vi "ALTS-2015 Scanner Driverv2.vi"(7 "Operation":T1, 8 "error in (no error)":errorcluster, 11 "Scanner 2?  (Scanner1)":bool) -> (0 "error out":errorcluster, 3 "Serial No":string)   [LabVIEW 2013]
doc: "Copyright © 2005, Soliton Technologies.\nAll rights reserved."
uses:
  <vilib>/Utility/file.llb/Read From Spreadsheet File (string).vi
  Controls/ALTS-2015 LV2GBL Options.ctl
  Controls/ALTS-2015 Scanner Driver Options.ctl
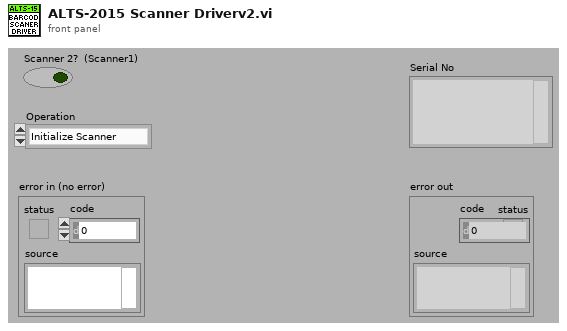
[diagram p1: front panel]
types:
  T1 = typedef "ALTS-2015 Scanner Driver Options.ctl" = enum16{"Initialize Scanner", "Read Scanner", "Close Scanner"}
  T2 = typedef "ALTS-2015 LV2GBL Options.ctl" = enum16{"Read all", "Write all"}
  T3 = typedef "ALTS-2015 INI Configuration Cluster.ctl" = cluster{"Application":cluster{"Rerun Count":i32, "Workorder No":string, "PLC Scanner":bool}, "Station Details":cluster{"Sensor Name 1":string, "Sensor Name 2":string, "Sensor Name 3":string, "Sensor Name 4":string, "Station1 Enable":bool, "Station2 Enable":bool, "Station3 Enable":bool, "Station4 Enable":bool}, "Database":cluster{"Database Connection Link":path, "Result Procedure":string, "User":string, "Password":string, "Prompt":bool, "Station 1 LT Result DB DSN Path":path, "Station 2 LT Result DB DSN Path":path, "Station 3 LT Result DB DSN Path":path, "Station 4 LT Result DB DSN Path":path, "AirLeakTestResult Procedure":string, "Serial Details Procedure":string}, "Simulation":cluster{"Simulate DAQ Hardware":bool, "Simulate Result DB Write":bool, "Simulate Scanner":bool, "Simulate OPC":bool, "Simulate Serial Details DB":bool, "Simulate Result DB":bool, "Simulate Scanner DB Path":path, "Simulate Serial Details DB Path":path, "Simulate Result DB Path":path}, "Barcode Scanner1":cluster{"Scanner IP":string, "Scanner Port":u16, "#Bytes to Read":i32, "Timeout_ms":i32}, "Barcode Scanner2":cluster{"Enabled?":bool, "Scanner IP":string, "Scanner Port":u16, "#Bytes to Read":i32}}
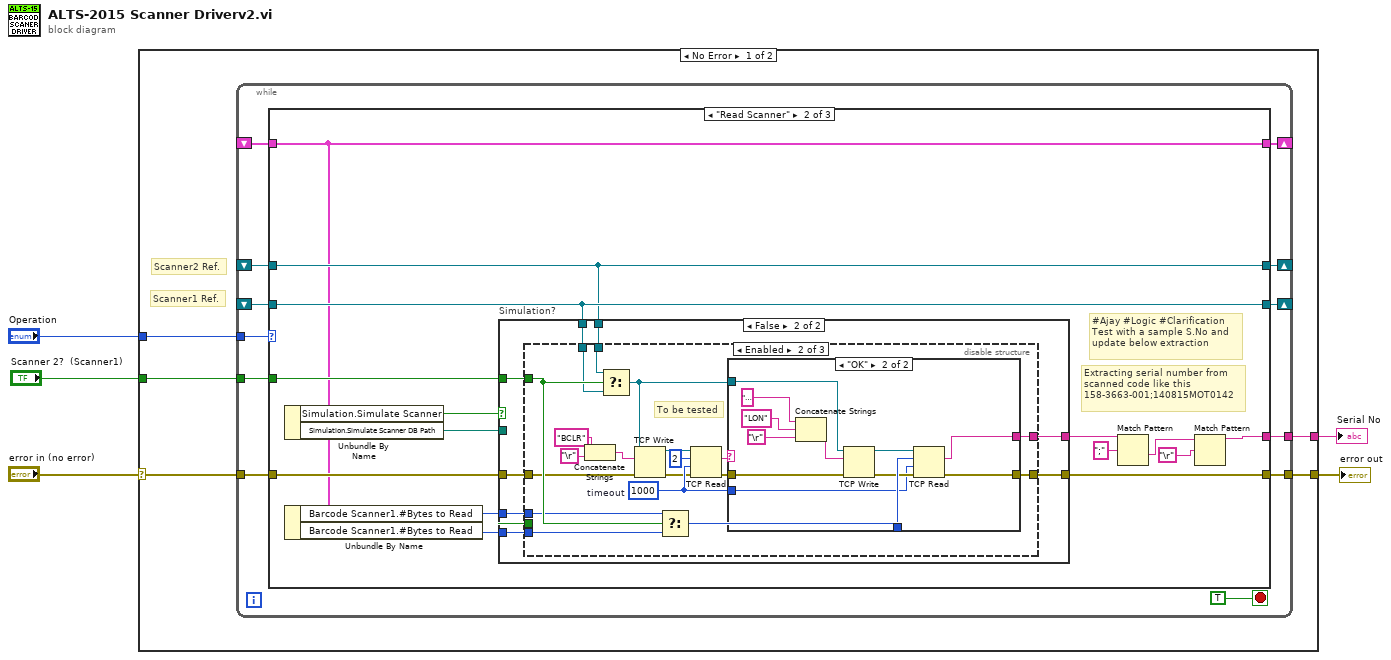
[diagram p0: block diagram]
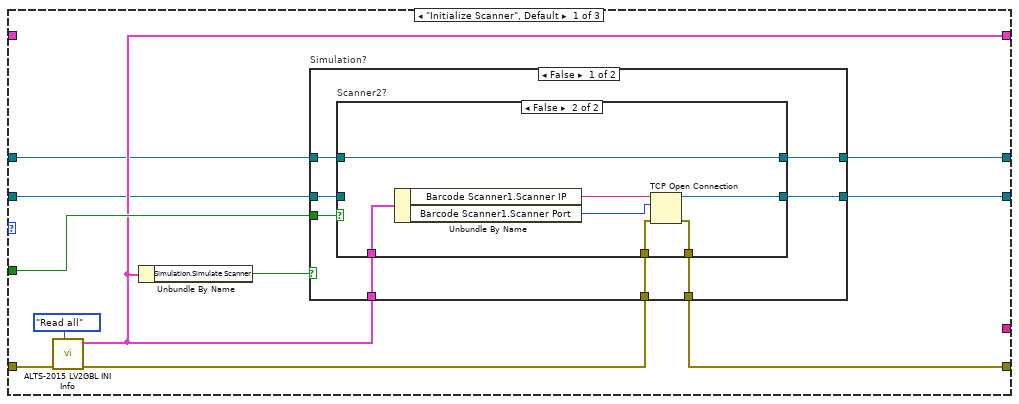
[diagram p2: hidden frame]
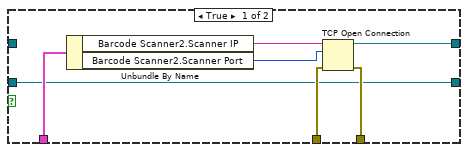
[diagram p3: hidden frame]
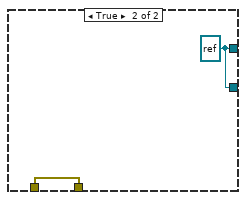
[diagram p4: hidden frame]
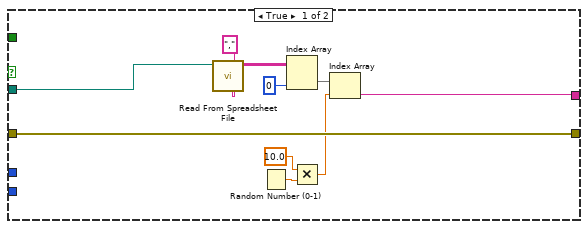
[diagram p5: hidden frame]
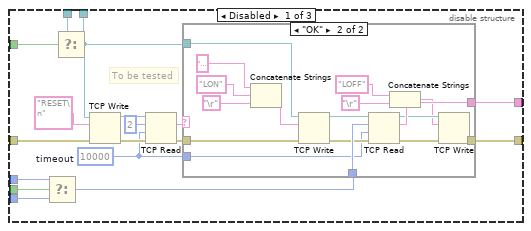
[diagram p6: hidden frame]
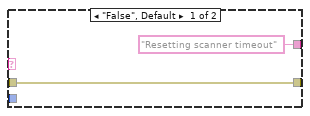
[diagram p7: hidden frame]
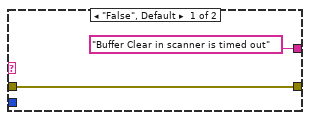
[diagram p8: hidden frame]
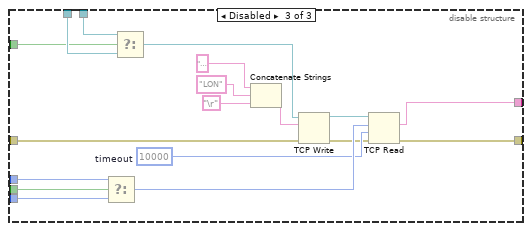
[diagram p9: hidden frame]
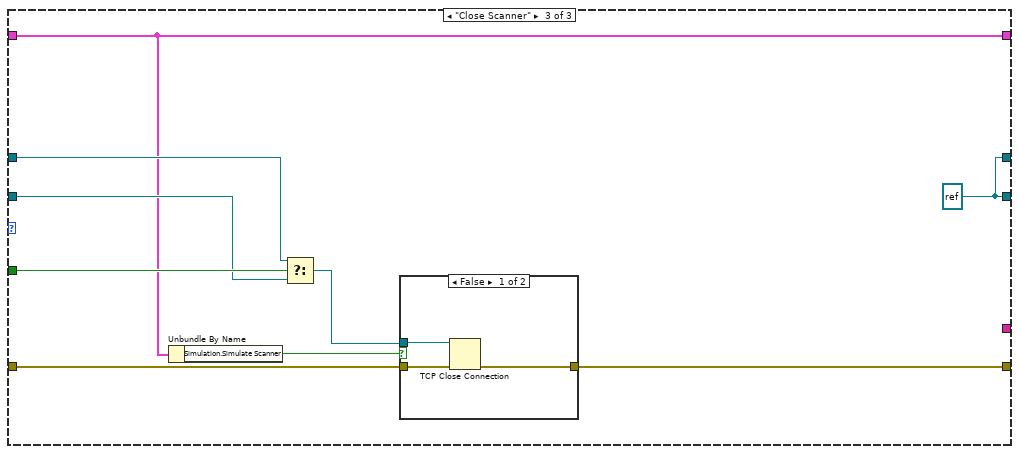
[diagram p10: hidden frame]
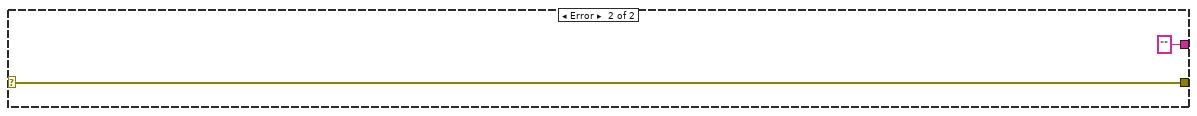
[diagram p12: hidden frame]
diagram:
  n1 = case shown="No Error" "error in (no error)" {
    selector: "error in (no error)" -> [w9 w191]
    tunnel: [w10 w191] -> w4
    tunnel: "Operation" -> [w8 _]
    tunnel: "Scanner 2?  (Scanner1)" -> [w7 _]
    tunnel: [w6 "" ("String")] -> w1
    frame No Error {
      # "Scanner1 Ref."
      # "Scanner2 Ref."
      n2 = while {
        tunnel: [w21] -> w10
        shift-right: [w20] -> _
        shift-left: _ -> [w19]
        tunnel: w9 -> [w18]
        tunnel: w8 -> [w17]
        tunnel: w7 -> [w16]
        shift-right: [w15] -> _
        shift-left: _ -> [w14]
        tunnel: [w13] -> w6
        shift-right: [w12] -> _
        shift-left: _ -> [w11]
        stop <- TRUE stop-if-true
        n3 = case shown="\"Read Scanner\"" w17 {
          tunnel: w18 -> [w33 w69 w184]
          tunnel: [w29 w72 w185] -> w21
          tunnel: [w31 w70 w178] -> w20
          tunnel: w19 -> [w23 w70 w180]
          tunnel: w16 -> [w32 w68 w182]
          tunnel: [w28 w71 w178] -> w15
          tunnel: w14 -> [w24 w71 w181]
          tunnel: [_ w59 _] -> w13
          tunnel: [w26 w58 w177] -> w12
          tunnel: w11 -> [_ w58 w177]
          frame "Initialize Scanner", Default {
            n4 = call "ALTS-2015 LV2GBL INI Info.vi"("Options"=ALTS-2015_LV2GBL_Options."Read all", "error in"=w33) -> ("error out"=w30:errorcluster, "Configuration Cluster Out"=w26:T3)  [unwired: 8 in]
            n5 = Unbundle By Name(w26) -> ("Simulation.Simulate Scanner"=w27:bool)
            n6 = case "Simulation?" shown="False" w27 {
              tunnel: w26 -> [w41 _]
              tunnel: w32 -> [w40 _]
              tunnel: [w39 w57] -> w31
              tunnel: w30 -> [w38 w56]
              tunnel: [w37 w56] -> w29
              tunnel: [w36 w57] -> w28
              tunnel: w24 -> [w35 _]
              tunnel: w23 -> [w34 _]
              frame False {
                n7 = case "Scanner2?" shown="False" w40 {
                  tunnel: w41 -> [w48 w55]
                  tunnel: [w43 w49] -> w39
                  tunnel: w38 -> [w45 w52]
                  tunnel: [w44 w51] -> w37
                  tunnel: [w42 w50] -> w36
                  tunnel: w35 -> [w42 _]
                  tunnel: w34 -> [_ w49]
                  frame True {
                    n8 = Unbundle By Name(w48) -> ("Barcode Scanner2.Scanner IP"=w47:string, "Barcode Scanner2.Scanner Port"=w46:u16)
                    n9 = TCP Open Connection(address=w47, remote port or service name=w46, error in (no error)=w45) -> (connection ID=w43:refnum<k5>, error out=w44:errorcluster)  [unwired: 2 in]
                  }
                  frame False {
                    n10 = Unbundle By Name(w55) -> ("Barcode Scanner1.Scanner IP"=w54:string, "Barcode Scanner1.Scanner Port"=w53:u16)
                    n11 = TCP Open Connection(address=w54, remote port or service name=w53, error in (no error)=w52) -> (connection ID=w50:refnum<k5>, error out=w51:errorcluster)  [unwired: 2 in]
                  }
                }
              }
              frame True {
                w57 = refnum<k5> refnum ("connection ID")
              }
            }
          }
          frame "Read Scanner" {
            # "#Ajay #Logic #Clarification\nTest with a sample S.No and\nupdate below extraction"
            # "Extracting serial number from \nscanned code like this \n158-3663-001;140815MOT0142"
            n12 = Unbundle By Name(w58) -> ("Simulation.Simulate Scanner"=w65:bool, "Simulation.Simulate Scanner DB Path"=w64:path)
            n13 = Unbundle By Name(w58) -> ("Barcode Scanner1.#Bytes to Read"=w67:i32, "Barcode Scanner1.#Bytes to Read"=w66:i32)
            n14 = case "Simulation?" shown="False" w65 {
              tunnel: [w82 w84] -> w72
              tunnel: w71 -> [_ w90]
              tunnel: w70 -> [_ w89]
              tunnel: [w73 w85] -> w63
              tunnel: w69 -> [w82 w88]
              tunnel: w68 -> [_ w83]
              tunnel: w67 -> [_ w87]
              tunnel: w66 -> [_ w86]
              tunnel: w64 -> [w74 _]
              frame True {
                n15 = call-poly <vilib>:"Read From Spreadsheet File.vi"("delimiter (\\t)"="," ("delimiter (\\t)"), "file path (dialog if empty)"=w74) -> ("all rows"=w77:string[][])  [unwired: 5 in, 4 out]
                n16 = Random Number (0-1)() -> (number: 0 to 1=w79:dbl)
                n17 = Index Array(array=w77, index (col)=0 ("disabled index (col)")) -> (element=w78:string[])  [unwired: 1 in]
                n18 = Multiply(x=10.0, y=w79) -> (x*y=w80:dbl)
                n19 = Index Array(array=w78, index=w80) -> (element=w73:string)
              }
              frame False {
                n20 = disable-structure shown="Enabled" {
                  disable-tunnel: w90 -> [w107 w130 w176]
                  disable-tunnel: w89 -> [w106 w129 w175]
                  disable-tunnel: w88 -> [w105 w131 w174]
                  disable-tunnel: w83 -> [w104 _ w173]
                  disable-tunnel: w87 -> [w103 w133 w172]
                  disable-tunnel: w86 -> [w102 w132 w171]
                  disable-tunnel: [w100 w127 w169] -> w85
                  disable-tunnel: [w99 w128 w162] -> w84
                  disable-tunnel: w83 -> [_ w134 _]
                  frame Disabled {
                    w94 = 10000  # timeout
                    # "To be tested"
                    n21 = Select(t=w103, s=w104, f=w102) -> (s? t:f=w101:i32)
                    n22 = Select(t=w106, s=w104, f=w107) -> (s? t:f=w97:refnum<k5>)
                    n23 = TCP Write(connection ID=w97, data in="RESET\n", error in (no error)=w105) -> (connection ID out=w92:refnum<k5>, error out=w98:errorcluster)  [unwired: 1 in, 1 out]
                    n24 = TCP Read(connection ID=w92, bytes to read=2, error in (no error)=w98, 9:w94) -> (data out=w91:string, error out=w95:errorcluster)  [unwired: 1 in, 1 out]
                    n25 = case shown="\"OK\"" w91 {
                      tunnel: w101 -> [_ w121]
                      tunnel: ["Resetting scanner timeout" ("data out") w119] -> w100
                      tunnel: [w109 w117] -> w99
                      tunnel: w97 -> [_ w112]
                      tunnel: w95 -> [w109 w111]
                      tunnel: w94 -> [_ w110]
                      frame "False", Default {
                      }
                      frame "OK" {
                        n26 = Concatenate Strings("\u001b", "LON", "\r" ("string")) -> (w125:string)
                        n27 = TCP Write(connection ID=w112, data in=w125, error in (no error)=w111) -> (connection ID out=w124:refnum<k5>, error out=w120:errorcluster)  [unwired: 2 out]
                        n28 = TCP Read(connection ID=w124, bytes to read=w121, error in (no error)=w120, 9:w110) -> (connection ID out=w116:refnum<k5>, data out=w119:string, error out=w122:errorcluster)  [unwired: 1 in]
                        n29 = Concatenate Strings("LOFF", "\r" ("string")) -> (w113:string)
                        n30 = TCP Write(connection ID=w116, data in=w113, error in (no error)=w122) -> (error out=w117:errorcluster)  [unwired: 1 in, 2 out]
                      }
                    }
                  }
                  frame Enabled {
                    w139 = 1000  # timeout
                    # "To be tested"
                    n31 = Concatenate Strings("BCLR", "\r" ("string")) -> (w145:string)
                    n32 = Select(t=w129, s=w134, f=w130) -> (s? t:f=w137:refnum<k5>)
                    n33 = TCP Write(connection ID=w137, data in=w145, error in (no error)=w131) -> (connection ID out=w141:refnum<k5>, error out=w136:errorcluster)  [unwired: 1 in, 1 out]
                    n34 = Select(t=w133, s=w134, f=w132) -> (s? t:f=w135:i32)
                    n35 = TCP Read(connection ID=w141, bytes to read=2, error in (no error)=w136, 9:w139) -> (data out=w142:string, error out=w138:errorcluster)  [unwired: 1 in, 1 out]
                    n36 = case shown="\"OK\"" w142 {
                      tunnel: w135 -> [_ w154]
                      tunnel: ["Buffer Clear in scanner is timed out" ("data out") w152] -> w127
                      tunnel: [w147 w155] -> w128
                      tunnel: w137 -> [_ w150]
                      tunnel: w138 -> [w147 w149]
                      tunnel: w139 -> [_ w148]
                      frame "False", Default {
                      }
                      frame "OK" {
                        n37 = Concatenate Strings("\u001b", "LON", "\r" ("string")) -> (w158:string)
                        n38 = TCP Write(connection ID=w150, data in=w158, error in (no error)=w149) -> (connection ID out=w157:refnum<k5>, error out=w153:errorcluster)  [unwired: 2 out]
                        n39 = TCP Read(connection ID=w157, bytes to read=w154, error in (no error)=w153, 9:w148) -> (data out=w152:string, error out=w155:errorcluster)  [unwired: 1 in, 1 out]
                      }
                    }
                  }
                  frame Disabled {
                    w167 = 10000  # timeout
                    n40 = Select(t=w172, s=w173, f=w171) -> (s? t:f=w170:i32)
                    n41 = Select(t=w175, s=w173, f=w176) -> (s? t:f=w168:refnum<k5>)
                    n42 = Concatenate Strings("\u001b", "LON", "\r" ("string")) -> (w165:string)
                    n43 = TCP Write(connection ID=w168, data in=w165, error in (no error)=w174) -> (connection ID out=w164:refnum<k5>, error out=w161:errorcluster)  [unwired: 2 out]
                    n44 = TCP Read(connection ID=w164, bytes to read=w170, error in (no error)=w161, 9:w167) -> (data out=w169:string, error out=w162:errorcluster)  [unwired: 1 in, 1 out]
                  }
                }
              }
            }
            n45 = Match Pattern(string=w63, regular expression=";") -> (after substring=w60:string)  [unwired: 1 in, 3 out]
            n46 = Match Pattern(string=w60, regular expression="\r" ("string")) -> (before substring=w59:string)  [unwired: 1 in, 3 out]
          }
          frame "Close Scanner" {
            w178 = refnum<k5> refnum ("connection ID")
            n47 = Unbundle By Name(w177) -> ("Simulation.Simulate Scanner"=w183:bool)
            n48 = Select(t=w180, s=w182, f=w181) -> (s? t:f=w179:refnum<k5>)
            n49 = case shown="False" w183 {
              tunnel: [w187 w189] -> w185
              tunnel: w179 -> [w186 _]
              tunnel: w184 -> [w188 w189]
              frame False {
                n50 = TCP Close Connection(connection ID=w186, error in (no error)=w188) -> (error out=w187:errorcluster)  [unwired: 1 in, 1 out]
              }
              frame True {
              }
            }
          }
        }
      }
    }
    frame Error {
    }
  }
  "error out" <- w4
  "Serial No" <- w1
